vi "testing commands.vi"() -> ()   [LabVIEW 2015, in "AguaClara Library.lvlib"]
uses:
  AguaClara Library.lvlib
  AutoCAD cmds.ctl
panel:
  in  "SourcePath":string
  in  "CExpressViewerControl":refnum<k7>(container)
  in  "Command":string="box 4 4 4\n_-view\n_swiso\n_shademode\nRealistic\n"
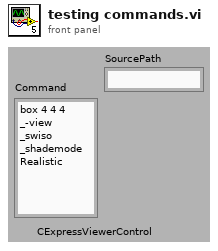
[diagram p1: front panel]
types:
  T1 = typedef "AguaClara Library.lvlib/AutoCAD cmds.ctl" = enum16{"Open AutoCAD", "New Document", "Send Command", "Send Command Array", "Close Doc", "Quit"}
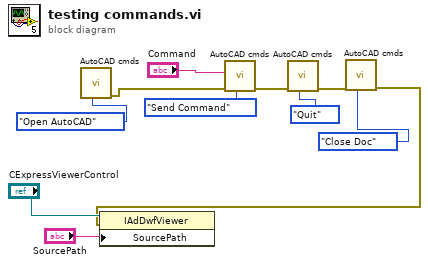
[diagram p0: block diagram]
diagram:
  n1 = call "AutoCAD cmds.vi"("AutoCAD cmd"=AutoCAD_cmds."Open AutoCAD") -> ("error out"=w5:errorcluster)  [unwired: 9 in, 1 out]
  n2 = call "AutoCAD cmds.vi"("AutoCAD cmd"=AutoCAD_cmds."Send Command", "error in (no error)"=w5, 10:"Command") -> ("error out"=w11:errorcluster)  [unwired: 7 in, 1 out]
  n3 = call "AutoCAD cmds.vi"("AutoCAD cmd"=AutoCAD_cmds."Quit", "error in (no error)"=w11) -> ("error out"=w10:errorcluster)  [unwired: 8 in, 1 out]
  n4 = call "AutoCAD cmds.vi"("AutoCAD cmd"=AutoCAD_cmds."Close Doc", "error in (no error)"=w10) -> ("error out"=w2:errorcluster)  [unwired: 8 in, 1 out]
  n5 = property class="IAdDwfViewer"(reference="CExpressViewerControl", error in=w2, "SourcePath"="SourcePath") -> ()  [unwired: 2 out]
